vi "conv-var-vers-MIF.vi"(7 "Variable":string) -> (1 "Obs (Ch)":string, 2 "MIF ?":bool, 3 "Obs.":T1)   [LabVIEW 2010, in "lv_04.lvlib"]
uses:
  lv_04.lvlib
  commandes/c_enum_obs.ctl
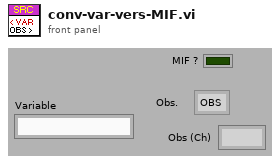
[diagram p1: front panel]
types:
  T1 = typedef "lv_04.lvlib/c_enum_obs.ctl" = enum16{"OBS", "MIF"}
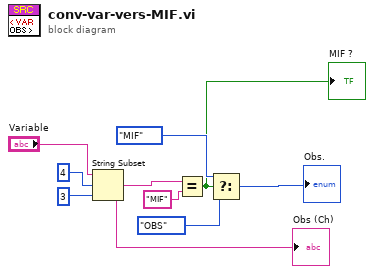
[diagram p0: block diagram]
diagram:
  n1 = String Subset(string="Variable", offset (0)=4, length (rest)=3 ("longueur (reste)")) -> (substring=w2:string)
  "Obs (Ch)" <- w2
  n2 = Equal?(x=w2, y="MIF") -> (x = y?=w1:bool)
  "MIF ?" <- w1
  n3 = Select(t=c_enum_obs."MIF" ("Obs."), s=w1, f=c_enum_obs."OBS" ("Obs.")) -> (s? t:f=→"Obs.":T1)
